vi "Ctor.vi"(8 "error in (no error)":errorcluster) -> (0 "error out":errorcluster, 3 "Manager out":refnum<class "Manager.lvclass">)   [LabVIEW 2020, in "Parallel Block.lvlib" / "Manager.lvclass"]
uses:
  Manager.lvclass
  Manager.lvclass/Manager.ctl
  Block/Block.lvclass
  Input/Input.lvclass
  Output/Output.lvclass
  Block State.ctl
  Block Map.ctl
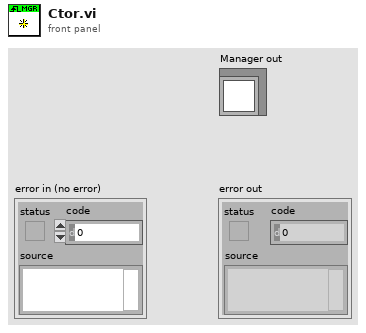
[diagram p1: front panel]
types:
  T1 = typedef "Parallel Block.lvlib/Manager.lvclass/Block Map.ctl" = map{refnum<class "Block.lvclass">, refnum<data-value>}
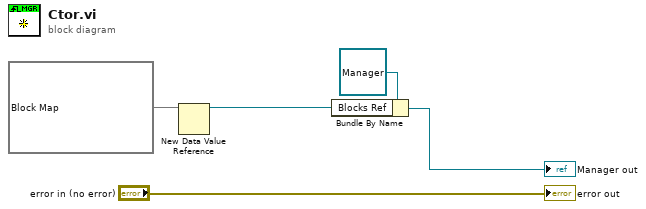
[diagram p0: block diagram]
diagram:
  n1 = New Data Value Reference(data value=T1 {} ("Block Map")) -> (data value reference=w1:refnum<data-value>)  [unwired: 1 in, 1 out]
  n2 = Bundle By Name(cluster=refnum<class "Manager.lvclass"> refnum ("Manager in"), "Blocks Ref"=w1) -> (→"Manager out":refnum<class "Manager.lvclass">)
  "error out" <- "error in (no error)"
